vi "UIRef.vi"(8 "error in":errorcluster, 11 "Logic Sequencer editor node in":refnum<class "Logic Sequencer editor node.lvclass">) -> (0 "error out":errorcluster, 2 "VI refnum":refnum<vi>, 3 "Logic Sequencer editor node out":refnum<class "Logic Sequencer editor node.lvclass">)   [LabVIEW 2013, in "Logic Sequencer editor node.lvclass"]
uses:
  Logic Sequencer editor node.lvclass
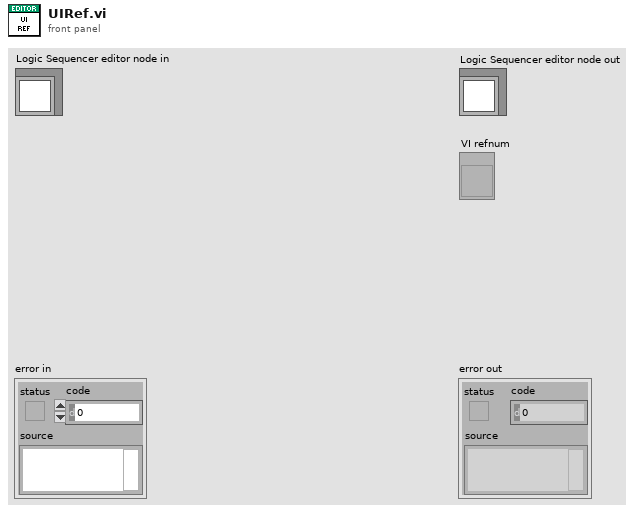
[diagram p1: front panel]
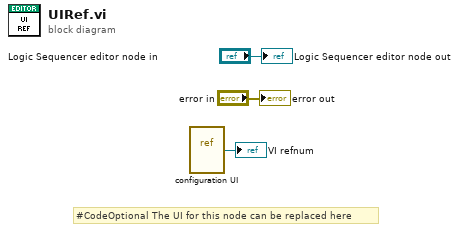
[diagram p0: block diagram]
diagram:
  # "#CodeOptional The UI for this node can be replaced here"
  n1 = vi-ref "configuration UI.vi"() -> (→"VI refnum":refnum<vi>)
  "error out" <- "error in"
  "Logic Sequencer editor node out" <- "Logic Sequencer editor node in"
